vi "Get_Characteristic_Velocity.vi"(9 "dt (bin width)":dbl, 11 "Velocity":dbl[](array[numeric])) -> (0 "Uo":dbl, 1 "Jet Frequency":dbl, 2 "Tb/T":dbl format="%_4g", 3 "Lo":dbl)   [LabVIEW 2011]
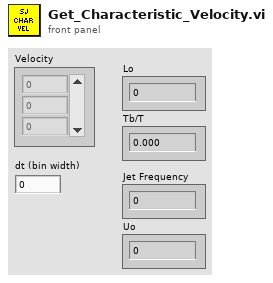
[diagram p1: front panel]
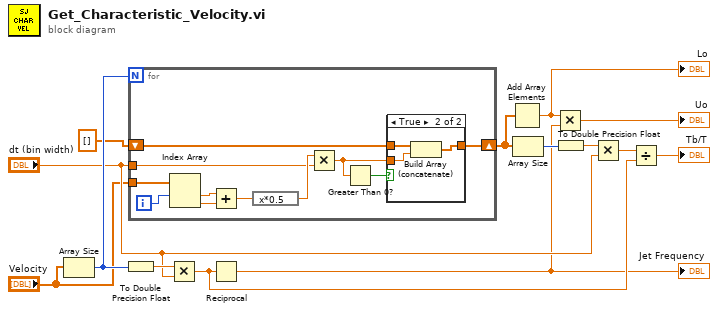
[diagram p0: block diagram]
diagram:
  n1 = Array Size(array="Velocity") -> (size(s)=w10:i32)
  n2 = To Double Precision Float(number=w10) -> (double precision float=w11:dbl)
  n3 = for {
    N: w10 -> [_]
    tunnel: "Velocity" -> [w25]
    tunnel: "dt (bin width)" -> [w20]
    shift-right: [w16] -> w14
    shift-left: dbl[] [] -> [w17]
    i -> [w15]
    n4 = Index Array(array=w25, index #1=w15) -> (element #1=w24:dbl, element #2=w23:dbl)  [unwired: 1 in]
    n5 = Add(x=w24, y=w23) -> (x+y=w22:dbl)
    n6 = expression code="x*0.5"(w22) -> (w21:dbl)
    n7 = Multiply(x=w21, y=w20) -> (x*y=w18:dbl)
    n8 = Greater Than 0?(x=w18) -> (x > 0?=w19:bool)
    n9 = case shown="True" w19 {
      tunnel: w18 -> [_ w29]
      tunnel: w17 -> [w26 w28]
      tunnel: [w26 w27] -> w16
      frame False {
      }
      frame True {
        n10 = Build Array (concatenate)(w28, w29) -> (w27:dbl[])
      }
    }
  }
  n11 = Multiply(x=w11, y="dt (bin width)") -> (x*y=w7:dbl)
  n12 = Reciprocal(x=w7) -> (1/x=w5:dbl)
  "Jet Frequency" <- w5
  n13 = Add Array Elements(numeric array=w14) -> (sum=w4:dbl)
  "Lo" <- w4
  n14 = Array Size(array=w14) -> (size(s)=w13:i32)
  n15 = Multiply(x=w4, y=w5) -> (x*y=→"Uo":dbl)
  n16 = To Double Precision Float(number=w13) -> (double precision float=w12:dbl)
  n17 = Multiply(x=w12, y="dt (bin width)") -> (x*y=w8:dbl)
  n18 = Divide(x=w8, y=w7) -> (x/y=→"Tb/T":dbl)
